vi "MainBaxterDemo.vi"() -> ()   [LabVIEW 2015]
doc: "Demos several of Baxter's features: joint command, read joint states, open and close grippers, nod head, read IR data."
uses:
  ROS/Code/JointPositions.ctl
  ROS/Code/Slider.ctl
  ROS/Code/SubVIs/BaxterSide.ctl
  BaxterVIs/RightGripper.vi
  BaxterVIs/LeftGripper.vi
  BaxterVIs/BothArmsPosition.vi
panel:
  out "Left Range Data":T1
  in  "Nod":bool
  in  "left gripper":u16(ring) items=["close"=0, "open"=100]
  in  "right gripper":u16(ring) items=["close"=0, "open"=100]
  in  "Parameters":T2 {"left_w2" scale=-180.0..180.0; "left_w1" scale=-180.0..180.0; "left_w0" scale=-180.0..180.0; "left_e1" scale=-180.0..180.0; "left_e0" scale=-180.0..180.0; "left_s1" scale=-180.0..180.0; "left_s0" scale=-180.0..180.0; "right_s1" scale=-180.0..180.0; "right_s0" scale=-180.0..180.0; "right_w2" scale=-180.0..180.0; "right_e1" scale=-180.0..180.0; "right_e0" scale=-180.0..180.0; "right_w0" scale=-180.0..180.0; "right_w1" scale=-180.0..180.0}
  out "Right Range Data":T1
  out "Joint States":T4(array[cluster])
  in  "stop":bool
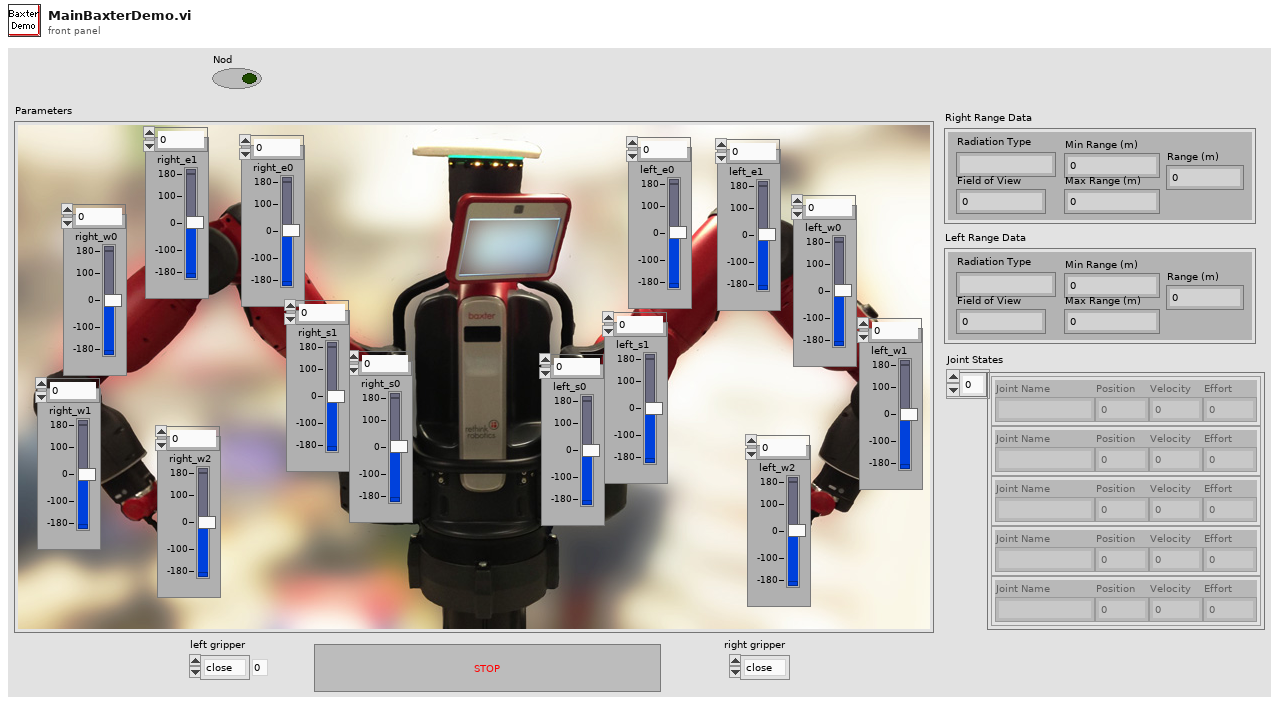
[diagram p1: front panel]
types:
  T1 = cluster{"Radiation Type":string, "Field of View":sgl, "Min Range (m)":sgl, "Max Range (m)":sgl, "Range (m)":sgl}
  T2 = typedef "JointPositions.ctl" = cluster{"left_e0":T3, "left_e1":T3, "left_s0":T3, "left_s1":T3, "left_w0":T3, "left_w1":T3, "left_w2":T3, "right_e0":T3, "right_e1":T3, "right_s0":T3, "right_s1":T3, "right_w0":T3, "right_w1":T3, "right_w2":T3}
  T3 = typedef "Slider.ctl" = dbl
  T4 = cluster{"Joint Name":string, "Position":dbl, "Velocity":dbl, "Effort":dbl}[]
  T5 = typedef "BaxterSide.ctl" = enum16{"left", "right"}
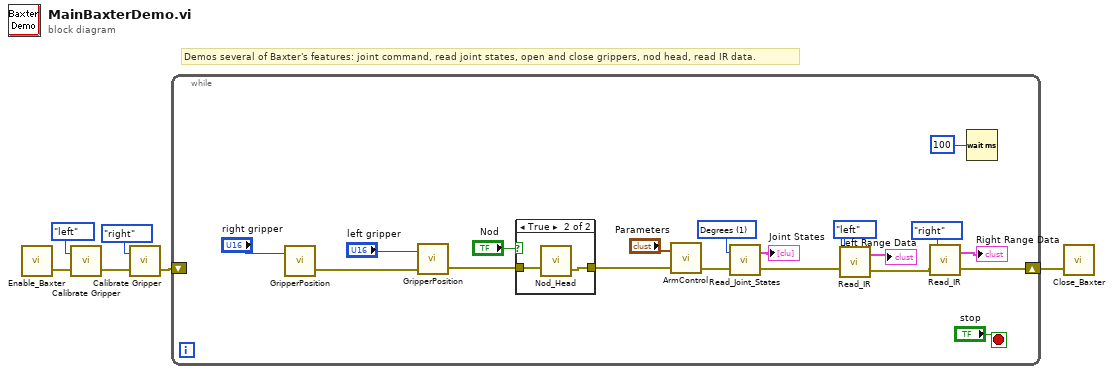
[diagram p0: block diagram]
diagram:
  # "Demos several of Baxter's features: joint command, read joint states, open and close grippers, nod head, read IR data."
  n1 = call "Enable_Baxter.vi"() -> ("error out"=w5:errorcluster)  [unwired: 4 in]
  n2 = call "Calibrate Gripper.vi"("error in"=w5, "Side"=BaxterSide."left") -> ("error out"=w6:errorcluster)  [unwired: 2 in]
  n3 = call "Calibrate Gripper.vi"("error in"=w6, "Side"=BaxterSide."right") -> ("error out"=w4:errorcluster)  [unwired: 2 in]
  n4 = while {
    shift-right: [w23] -> w1
    shift-left: w4 -> [_]
    stop <- "stop" stop-if-true
    w20 = u16 1 items=["Radians", "Degrees"] ("Units (Rad)")
    n5 = call-poly "GripperPosition.vi"("Desired Position"="right gripper") -> ("error out"=w10:errorcluster)  [unwired: 3 in]
    n6 = call-poly "GripperPosition.vi"("error in"=w10, "Desired Position"="left gripper") -> ("error out"=w13:errorcluster)  [unwired: 2 in]
    n7 = case shown="True" "Nod" {
      tunnel: [w26 w28] -> w8
      tunnel: w13 -> [w26 w27]
      frame False {
      }
      frame True {
        n8 = call "Nod_Head.vi"("error in"=w27) -> ("error out"=w28:errorcluster)  [unwired: 3 in]
      }
    }
    n9 = call-poly "ArmControl.vi"("error in"=w8, "Parameters"="Parameters") -> ("error out"=w7:errorcluster)  [unwired: 2 in]
    n10 = call "Read_Joint_States.vi"("error in"=w7, "Units (deg)"=w20) -> ("error out"=w17:errorcluster, "Joint States"=→"Joint States":T4)  [unwired: 1 in]
    n11 = call "Read_IR.vi"("error in"=w17, "Side"=BaxterSide."left") -> ("error out"=w16:errorcluster, "Range Data"=→"Left Range Data":T1)  [unwired: 1 in]
    n12 = call "Read_IR.vi"("error in"=w16, "Side"=BaxterSide."right") -> ("error out"=w23:errorcluster, "Range Data"=→"Right Range Data":T1)  [unwired: 1 in]
    n13 = Wait (ms)(milliseconds to wait=u32 100) -> ()  [unwired: 1 out]
  }
  n14 = call "Close_Baxter.vi"("error in"=w1) -> ()  [unwired: 3 in, 1 out]
